vi "Get Display String.vi"(11 "FP LT in":refnum<class "FP LT.lvclass">) -> (2 "Display String":string)   [LabVIEW 2018, in "FP LT.lvclass"]
uses:
  FP LT.lvclass
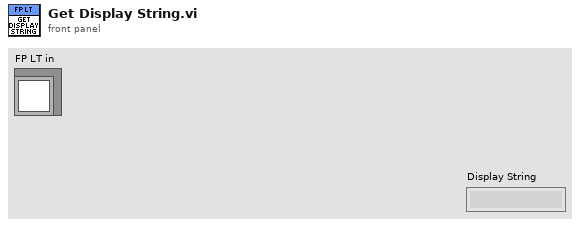
[diagram p1: front panel]
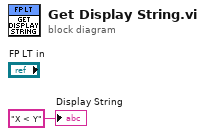
[diagram p0: block diagram]
diagram:
  "Display String" <- "X < Y" ("Display String")
